vi "Merge Maps Helper.vi"(9 "map in":map{string, dbl}(c390), 11 "Data Table in":map{string, dbl}(c390)) -> (3 "Data Table out":map{string, dbl}(c390))   [LabVIEW 2024, in "FlexiFlowInterfaceCH2.lvlib"]
uses:
  FlexiFlowInterfaceCH2.lvlib
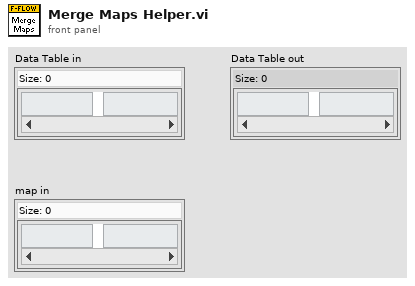
[diagram p1: front panel]
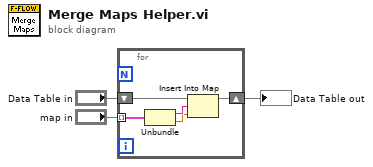
[diagram p0: block diagram]
diagram:
  n1 = for {
    shift-right: [w7] -> w3
    shift-left: "Data Table in" -> [w8]
    tunnel: "map in" -> [w6] mode=indexing
    n2 = Unbundle(w6) -> (w5:string, w4:dbl)
    n3 = Insert Into Map(map in=w8, key=w5, value=w4) -> (map out=w7:map{string, dbl})  [unwired: 2 out]
  }
  "Data Table out" <- w3
